vi "3D Cartesian Coordinate Rotation (Euler) (Array).vi"(6 "rotation order":T1=10 items=["X-Y-Z", "X-Z-Y", "Y-X-Z", "Y-Z-X", "Z-X-Y", "Z-Y-X", "X-Y-X", "X-Z-X", "Y-X-Y", "Y-Z-Y", "Z-X-Z", "Z-Y-Z"], 8 "Euler Angles":cluster{"phi":dbl, "theta":dbl, "psi":dbl}, 9 "Z":dbl[](array[numeric]), 10 "Y":dbl[](array[numeric]), 11 "X":dbl[](array[numeric])) -> (0 "error":i32, 1 "Z Out":dbl[](array[numeric]), 2 "Y Out":dbl[](array[numeric]), 3 "X Out":dbl[](array[numeric]))   [LabVIEW 2017, in "NI_AALPro.lvlib"]
doc: "Rotates a three-dimensional Cartesian coordinate in the counterclockwise direction using the Euler angles method. Wire data to the <B>X</B> input to determine the polymorphic instance to use or manually select the instance."
uses:
  NI_AALPro.lvlib
  Euler Rotation Order.ctl
  lvanlys.dll
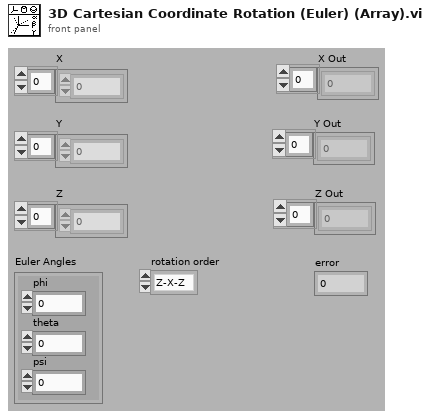
[diagram p1: front panel]
types:
  T1 = typedef "NI_AALPro.lvlib/Euler Rotation Order.ctl" = u16
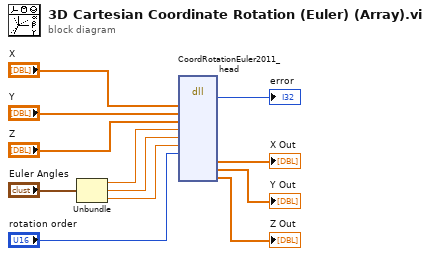
[diagram p0: block diagram]
diagram:
  n1 = Unbundle("Euler Angles") -> ("phi"=w4:dbl, "theta"=w3:dbl, "psi"=w2:dbl)
  n2 = dll-call lib="C:/Program Files/National Instruments/LabVIEW 2017/resource/lvanlys.*" fn="CoordRotationEuler2011_head"("X"="X", "Y"="Y", "Z"="Z", "phi"=w4, "theta"=w3, "psi"=w2, "rotateOrder"="rotation order") -> ("return type"=→"error":i32, "Xout"=→"X Out":dbl[], "Yout"=→"Y Out":dbl[], "Zout"=→"Z Out":dbl[])  [unwired: 13 in, 2 out]
